vi "Set Motors.vi"(0 "UniCyRO_Host_Sim in":refnum<class "UniCyRO_Host_Sim.lvclass">, 5 "Gyro Motor ccw velocity (rad/s)":dbl, 7 "Drive Motor ccw velocity (rad/s)":dbl, 9 "Torsion Motor ccw velocity (rad/s)":dbl, 11 "error in (no error)":errorcluster) -> (4 "UniCyRO_Host_Sim out":refnum<class "UniCyRO_Host_Sim.lvclass">, 15 "error out":errorcluster)   [LabVIEW 2012, in "UniCyRO.lvlib" / "UniCyRO_Host_Sim.lvclass"]
uses:
  UniCyRO_Host_Sim.lvclass
  UniCyRO_Host_Sim.lvclass/UniCyRO_Host_Sim.ctl
  <instrlib>/DC Motor Controller/HAIOL/DC Motor Controller.lvclass
  <vilib>/robotics/Utilities/NI_Robotics Utilities.lvlib
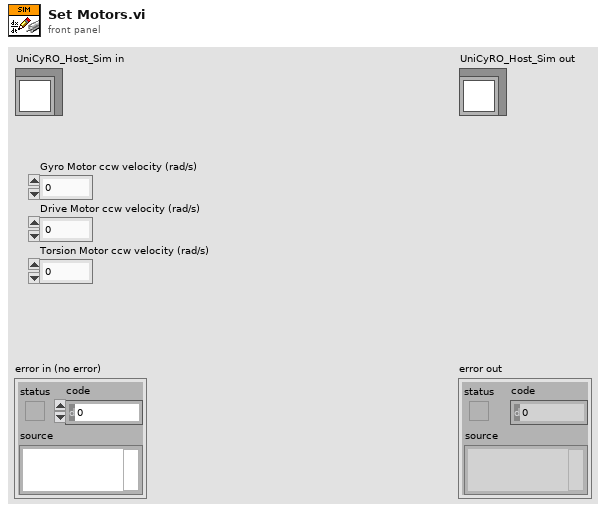
[diagram p1: front panel]
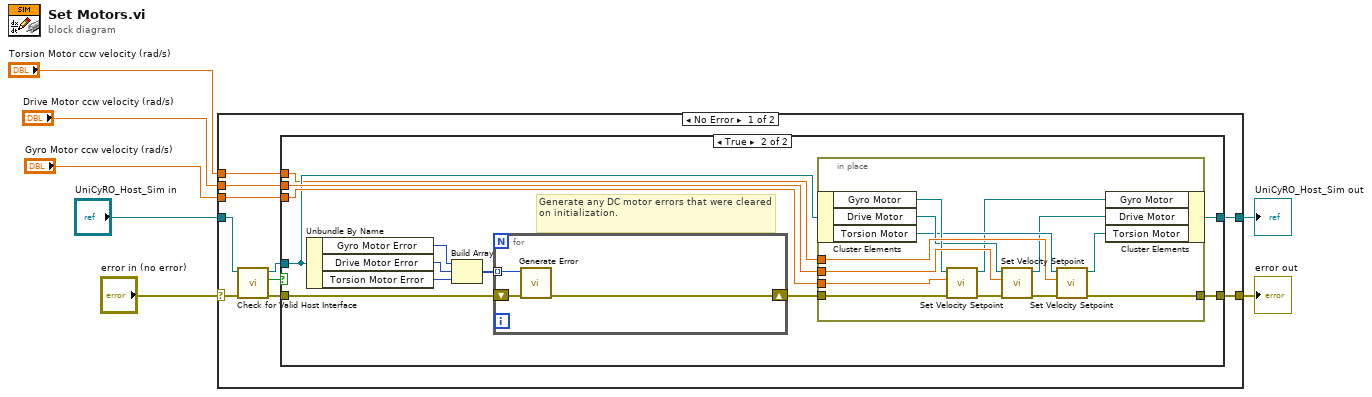
[diagram p0: block diagram]
diagram:
  n1 = case shown="No Error" "error in (no error)" {
    selector: "error in (no error)" -> [w10 w49]
    tunnel: [w16 w49] -> w2
    tunnel: [w17 w48] -> w4
    tunnel: "UniCyRO_Host_Sim in" -> [w11 w48]
    tunnel: "Gyro Motor ccw velocity (rad/s)" -> [w15 _]
    tunnel: "Drive Motor ccw velocity (rad/s)" -> [w14 _]
    tunnel: "Torsion Motor ccw velocity (rad/s)" -> [w13 _]
    frame No Error {
      n2 = call "Check for Valid Host Interface.vi"("error in (no error)"=w10, "UniCyRO_Host_Sim in"=w11) -> ("error out"=w9:errorcluster, "valid?"=w8:bool, "UniCyRO_Host_Sim out"=w12:refnum<class "UniCyRO_Host_Sim.lvclass">)  [unwired: 7 in]
      n3 = case shown="True" w8 {
        tunnel: [w19 w31] -> w17
        tunnel: [w18 w30] -> w16
        tunnel: w15 -> [_ w29]
        tunnel: w14 -> [_ w28]
        tunnel: w9 -> [w18 w21]
        tunnel: w12 -> [w19 w27]
        tunnel: w13 -> [_ w22]
        frame False {
        }
        frame True {
          # "Generate any DC motor errors that were cleared on initialization."
          n4 = Unbundle By Name(w27) -> ("Gyro Motor Error"=w25:i32, "Drive Motor Error"=w24:i32, "Torsion Motor Error"=w23:i32)
          n5 = Build Array(w25, w24, w23) -> (w26:i32[])
          n6 = for {
            shift-right: [w33] -> w20
            shift-left: w21 -> [w34]
            tunnel: w26 -> [w32] mode=indexing
            n7 = call <vilib>:"Generate Error.vi"("error in (no error)"=w34, "code"=w32) -> ("error out"=w33:errorcluster)  [unwired: 9 in]
          }
          n8 = in-place {
            in-place-border: [w42] -> w30
            in-place-border: w20 -> [w46]
            in-place-border: w29 -> [w45]
            in-place-border: w28 -> [w44]
            in-place-border: w22 -> [w41]
            n9 = in-place-cluster #1(w27) -> ("Gyro Motor"=w40:refnum<class "DC Motor Controller.lvclass">, "Drive Motor"=w39:refnum<class "DC Motor Controller.lvclass">, "Torsion Motor"=w38:refnum<class "DC Motor Controller.lvclass">)
            n10 = call-dynamic "Set Velocity Setpoint.vi"("error in (no error)"=w46, "CCW Velocity (0 rad/s)"=w45, "DC Motor Controller in"=w40) -> ("error out"=w47:errorcluster, "DC Motor Controller out"=w37:refnum<class "DC Motor Controller.lvclass">)  [unwired: 7 in]
            n11 = call-dynamic "Set Velocity Setpoint.vi"("error in (no error)"=w47, "CCW Velocity (0 rad/s)"=w44, "DC Motor Controller in"=w39) -> ("error out"=w43:errorcluster, "DC Motor Controller out"=w36:refnum<class "DC Motor Controller.lvclass">)  [unwired: 7 in]
            n12 = call-dynamic "Set Velocity Setpoint.vi"("error in (no error)"=w43, "CCW Velocity (0 rad/s)"=w41, "DC Motor Controller in"=w38) -> ("error out"=w42:errorcluster, "DC Motor Controller out"=w35:refnum<class "DC Motor Controller.lvclass">)  [unwired: 7 in]
            n13 = in-place-cluster #1("Gyro Motor"=w37, "Drive Motor"=w36, "Torsion Motor"=w35) -> (w31:refnum<class "UniCyRO_Host_Sim.lvclass">)
          }
        }
      }
    }
    frame Error {
    }
  }
  "error out" <- w2
  "UniCyRO_Host_Sim out" <- w4
